vi "(Var) Get_HVPS_2.vi"() -> ()   [LabVIEW 2017]
panel:
  out "G2. Q Stop":bool=TRUE
  out "G2. Stop":bool=TRUE
  out "G2. Start":bool=TRUE
  out "G2. Error ?":bool
  out "G2. mA":dbl
  out "G2. KV":dbl
  out "G2. Read Mode":string
  out "G2. Read HV":string
  out "G2. Read State":string
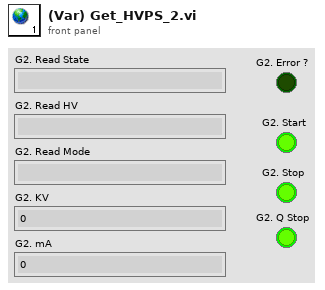
[diagram p1: front panel]
diagram:
